vi "CRYRub & Buzz Spreading.vi"(8 "number":i32, 9 "Pp[k]":dbl[](array[numeric]), 10 "Version":i32, 11 "Real matrix":dbl[][](array[numeric])) -> (3 "E2[k]":dbl[](array[numeric]))   [LabVIEW 2013]
panel:
  out "Su[k]":dbl[](array[numeric])
  out "Eline[j,k]":dbl[][](array[numeric])
  out "Eline1[j,k]":dbl[][](array[numeric])
  out "Sl[k]":dbl[](array[numeric])
  out "NormSP[k]":dbl[](array[numeric])
  out "L[k]":dbl[](array[numeric])
  in  "res":dbl
  out "Su[k]":dbl[](array[numeric])
  out "Eline[j,k]":dbl[][](array[numeric])
  out "Eline1[j,k]":dbl[][](array[numeric])
  out "Sl[k]":dbl[](array[numeric])
  out "L[k]":dbl[](array[numeric])
  in  "res":dbl
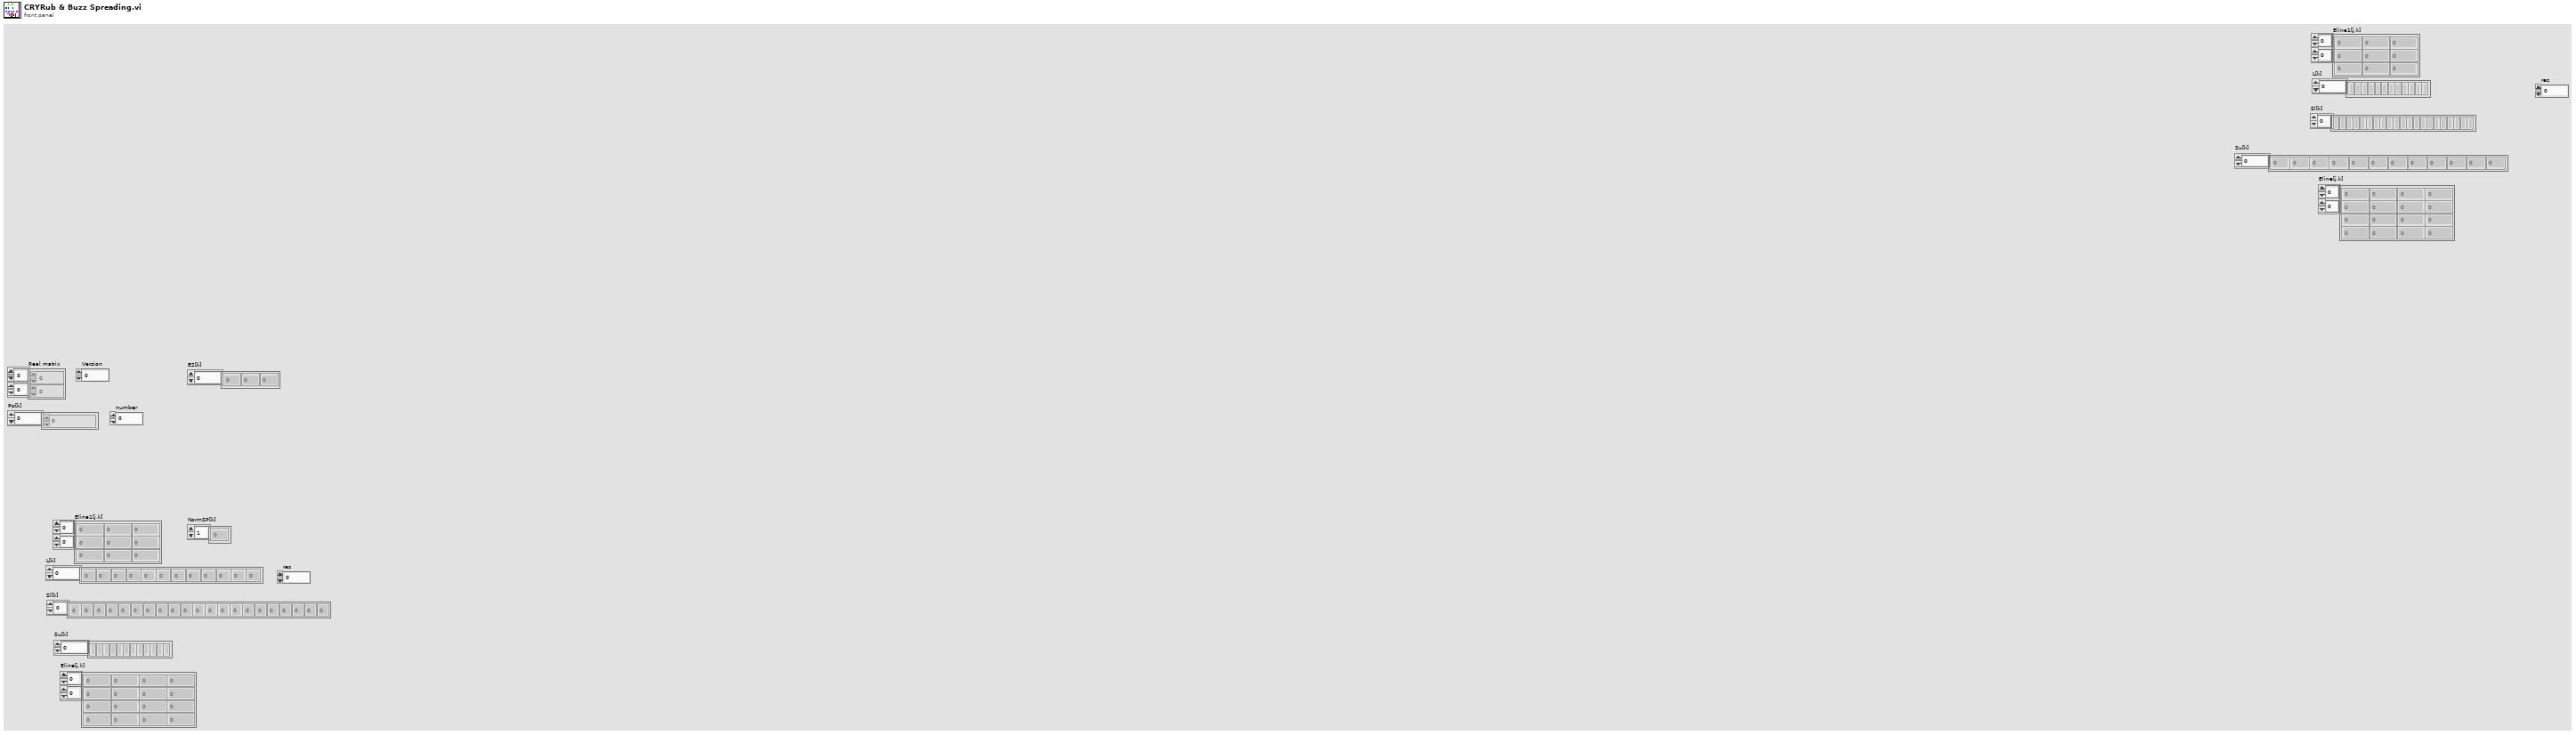
[diagram p1: front panel]
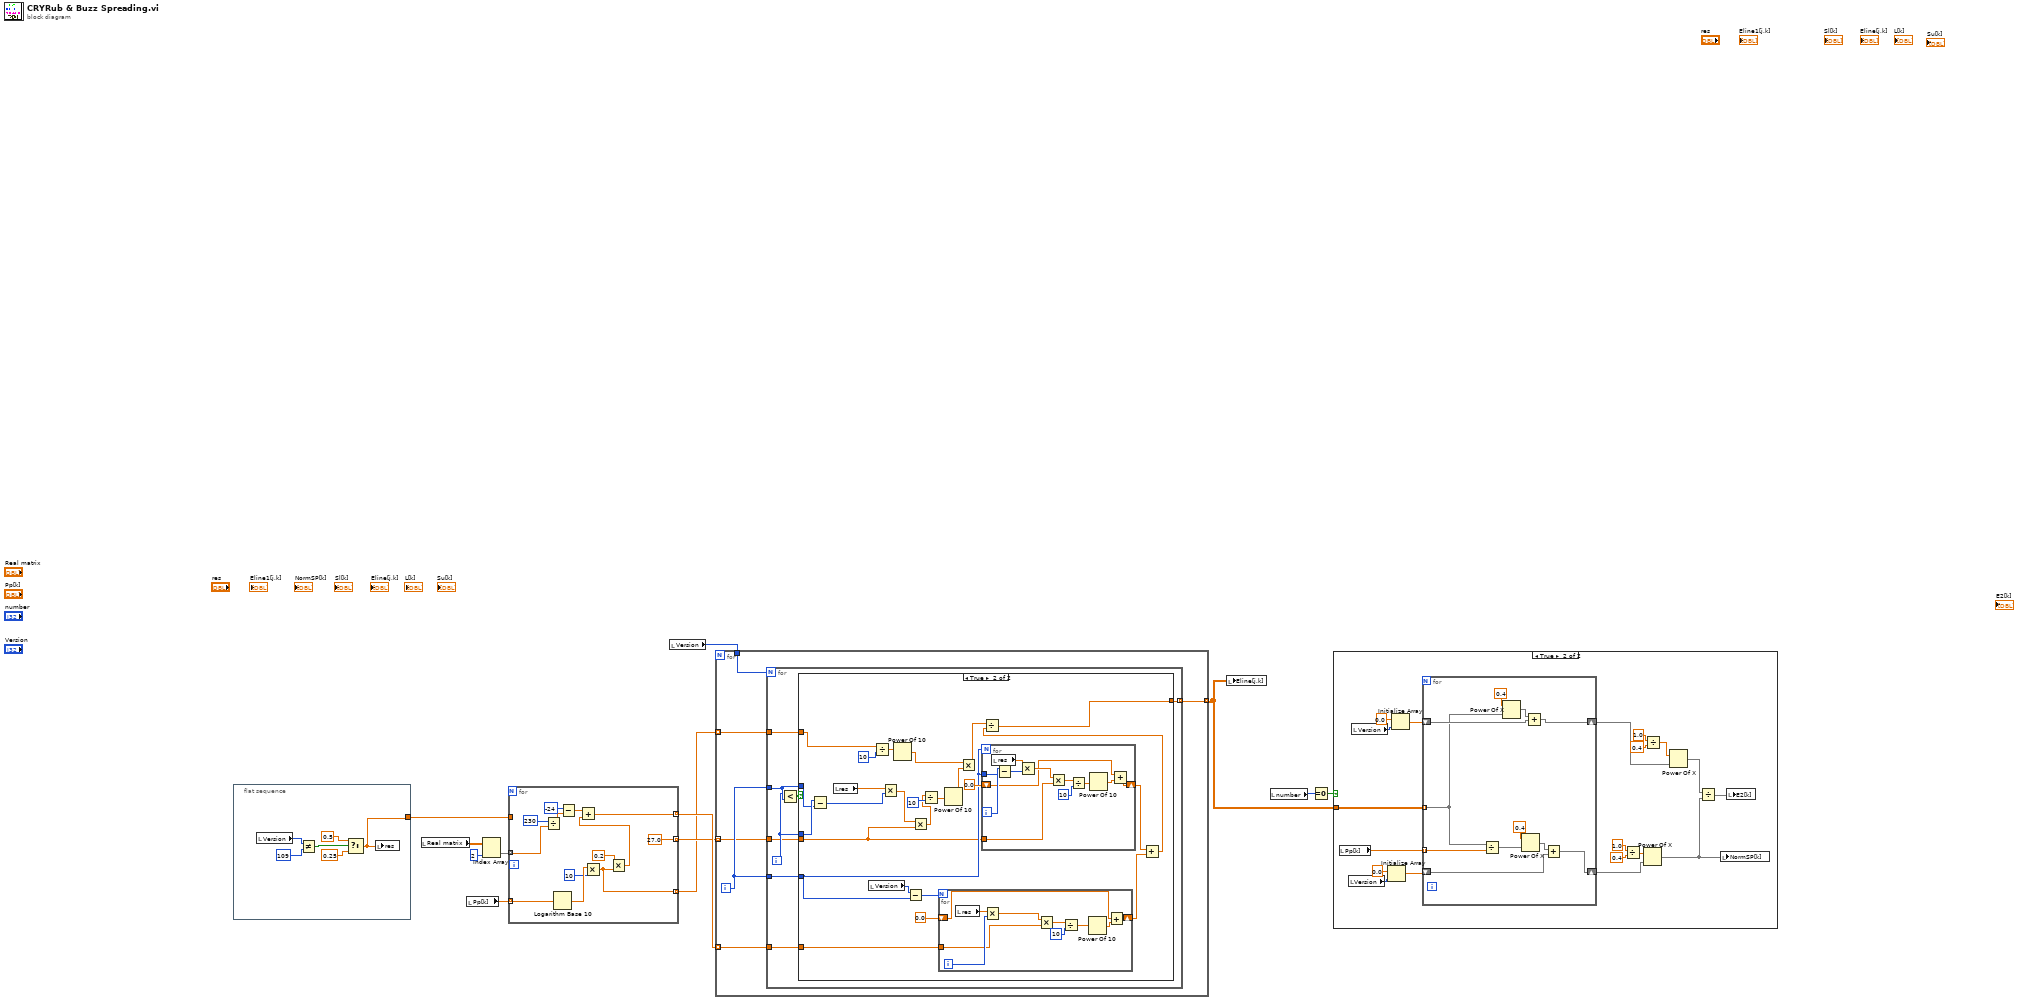
[diagram p0: block diagram]
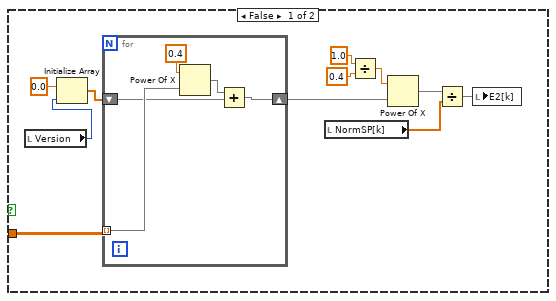
[diagram p2: hidden frame]
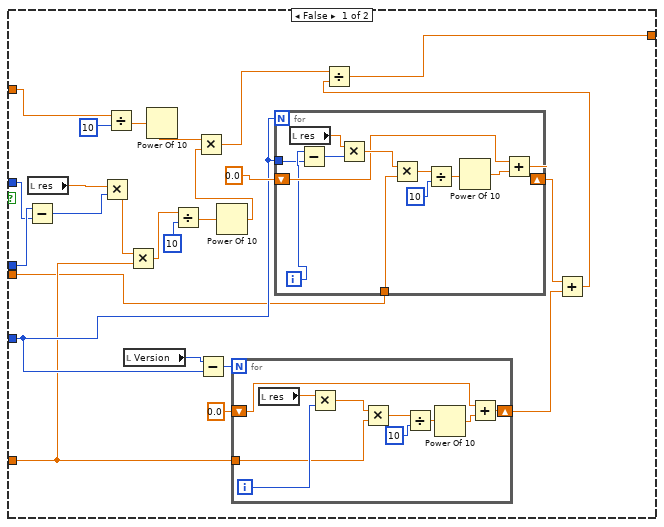
[diagram p3: hidden frame]
diagram:
  n1 = flat-sequence {
    tunnel: [w13] -> w3
    frame #0 {
      n2 = local read "Version"() -> (w17:i32)
      n3 = Not Equal?(x=w17, y=109) -> (x != y?=w16:bool)
      n4 = Select(t=0.5, s=w16, f=0.25) -> (s? t:f=w13:dbl)
      n5 = local write "res"(w13) -> ()
    }
  }
  n6 = local read "Real matrix"() -> (w8:dbl[][])
  n7 = local read "Pp[k]"() -> (w1:dbl[])
  n8 = Index Array(array=w8, index (col)=2 ("disabled index (col)")) -> (element=w6:dbl[])  [unwired: 1 in]
  n9 = for {
    tunnel: w1 -> [w23] mode=indexing
    tunnel: w6 -> [w19] mode=indexing
    tunnel: [w22] -> w10 mode=indexing
    tunnel: [27.0] -> w9 mode=indexing
    tunnel: [w20] -> w2 mode=indexing
    tunnel: w3 -> [_]
    n10 = Divide(x=230, y=w19) -> (x/y=w28:dbl)
    n11 = Logarithm Base 10(1:w23) -> (0:w31:dbl)
    n12 = Subtract(x=-24, y=w28) -> (x-y=w25:dbl)
    n13 = Multiply ("Multiply.vi")(x=w31, y=10) -> (x*y=w20:dbl)
    n14 = Multiply ("Multiply.vi")(x=0.2, y=w20) -> (x*y=w24:dbl)
    n15 = Add ("Add.vi")(x=w25, y=w24) -> (x+y=w22:dbl)
  }
  n16 = local read "Version"() -> (w11:i32)
  n17 = for {
    tunnel: w11 -> [w37]
    tunnel: w10 -> [w36] mode=indexing
    tunnel: w2 -> [w34] mode=indexing
    tunnel: [w32] -> w12 mode=indexing
    tunnel: w9 -> [w33] mode=indexing
    i -> [w35]
    n18 = for {
      N: w37 -> [_]
      tunnel: w35 -> [w44]
      tunnel: w35 -> [w43]
      tunnel: w36 -> [w41]
      tunnel: w34 -> [w40]
      tunnel: [w39] -> w32 mode=indexing
      tunnel: w33 -> [w38]
      i -> [w42]
      n19 = Less?(x=w42, y=w44) -> (x < y?=w45:bool)
      n20 = case shown="True" w45 {
        tunnel: w44 -> [w59 w105]
        tunnel: w42 -> [w60 w116]
        tunnel: w43 -> [w52 w100]
        tunnel: w41 -> [w48 w94]
        tunnel: w40 -> [w50 w97]
        tunnel: [w49 w96] -> w39
        tunnel: w38 -> [w47 w95]
        frame False {
          n21 = Subtract(x=w60, y=w59) -> (x-y=w69:i32)
          n22 = local read "res"() -> (w46:dbl)
          n23 = Multiply(x=w46, y=w69) -> (x*y=w55:dbl)
          n24 = Divide(x=w50, y=10) -> (x/y=w65:dbl)
          n25 = local read "Version"() -> (w51:i32)
          n26 = Multiply ("Multiply.vi")(x=w55, y=w48) -> (x*y=w54:dbl)
          n27 = Power Of 10(x=w65) -> (10^x=w64:dbl)
          n28 = Divide(x=w54, y=10) -> (x/y=w67:dbl)
          n29 = Subtract(x=w51, y=w52) -> (x-y=w63:i32)
          n30 = Power Of 10(x=w67) -> (10^x=w66:dbl)
          n31 = Multiply ("Multiply.vi")(x=w64, y=w66) -> (x*y=w61:dbl)
          n32 = for {
            N: w63 -> [_]
            shift-right: [w74] -> w62
            shift-left: 0.0 ("10^x") -> [w71]
            tunnel: w48 -> [w73]
            i -> [w80]
            n33 = local read "res"() -> (w72:dbl)
            n34 = Multiply ("Multiply.vi")(x=w72, y=w80) -> (x*y=w79:dbl)
            n35 = Multiply ("Multiply.vi")(x=w79, y=w73) -> (x*y=w78:dbl)
            n36 = Divide(x=w78, y=10) -> (x/y=w76:dbl)
            n37 = Power Of 10(x=w76) -> (10^x=w75:dbl)
            n38 = Add ("Add.vi")(x=w71, y=w75) -> (x+y=w74:dbl)
          }
          n39 = for {
            N: w52 -> [_]
            tunnel: w52 -> [w83]
            shift-right: [w85] -> w58
            shift-left: 0.0 ("10^x") -> [w86]
            tunnel: w47 -> [w82]
            i -> [w84]
            n40 = local read "res"() -> (w81:dbl)
            n41 = Subtract(x=w84, y=w83) -> (x-y=w92:i32)
            n42 = Multiply ("Multiply.vi")(x=w81, y=w92) -> (x*y=w91:dbl)
            n43 = Multiply ("Multiply.vi")(x=w91, y=w82) -> (x*y=w90:dbl)
            n44 = Divide(x=w90, y=10) -> (x/y=w88:dbl)
            n45 = Power Of 10(x=w88) -> (10^x=w87:dbl)
            n46 = Add ("Add.vi")(x=w86, y=w87) -> (x+y=w85:dbl)
          }
          n47 = Add ("Add.vi")(x=w58, y=w62) -> (x+y=w53:dbl)
          n48 = Divide(x=w61, y=w53) -> (x/y=w49:dbl)
        }
        frame True {
          n49 = Subtract(x=w116, y=w105) -> (x-y=w115:i32)
          n50 = local read "res"() -> (w93:dbl)
          n51 = local read "Version"() -> (w98:i32)
          n52 = Divide(x=w97, y=10) -> (x/y=w111:dbl)
          n53 = Multiply(x=w93, y=w115) -> (x*y=w104:dbl)
          n54 = Power Of 10(x=w111) -> (10^x=w110:dbl)
          n55 = Subtract(x=w98, y=w100) -> (x-y=w109:i32)
          n56 = Multiply ("Multiply.vi")(x=w104, y=w95) -> (x*y=w103:dbl)
          n57 = Divide(x=w103, y=10) -> (x/y=w113:dbl)
          n58 = for {
            N: w109 -> [_]
            shift-right: [w121] -> w107
            shift-left: 0.0 -> [w120]
            tunnel: w94 -> [w119]
            i -> [w127]
            n59 = local read "res"() -> (w118:dbl)
            n60 = Multiply(x=w118, y=w127) -> (x*y=w126:dbl)
            n61 = Multiply ("Multiply.vi")(x=w126, y=w119) -> (x*y=w125:dbl)
            n62 = Divide(x=w125, y=10) -> (x/y=w123:dbl)
            n63 = Power Of 10(x=w123) -> (10^x=w122:dbl)
            n64 = Add ("Add.vi")(x=w120, y=w122) -> (x+y=w121:dbl)
          }
          n65 = Power Of 10(x=w113) -> (10^x=w112:dbl)
          n66 = Multiply ("Multiply.vi")(x=w110, y=w112) -> (x*y=w106:dbl)
          n67 = for {
            N: w100 -> [_]
            tunnel: w100 -> [w138]
            shift-right: [w133] -> w108
            shift-left: 0.0 -> [w130]
            tunnel: w95 -> [w129]
            i -> [w139]
            n68 = local read "res"() -> (w128:dbl)
            n69 = Subtract(x=w139, y=w138) -> (x-y=w137:i32)
            n70 = Multiply(x=w128, y=w137) -> (x*y=w136:dbl)
            n71 = Multiply ("Multiply.vi")(x=w136, y=w129) -> (x*y=w135:dbl)
            n72 = Divide(x=w135, y=10) -> (x/y=w132:dbl)
            n73 = Power Of 10(x=w132) -> (10^x=w131:dbl)
            n74 = Add ("Add.vi")(x=w130, y=w131) -> (x+y=w133:dbl)
          }
          n75 = Add ("Add.vi")(x=w108, y=w107) -> (x+y=w101:dbl)
          n76 = Divide(x=w106, y=w101) -> (x/y=w96:dbl)
        }
      }
    }
  }
  n77 = local write "Eline[j,k]"(w12) -> ()
  n78 = local read "number"() -> (w5:i32)
  n79 = Equal To 0?(x=w5) -> (x = 0?=w4:bool)
  n80 = case shown="True" w4 {
    tunnel: w12 -> [w150 w174]
    frame False {
      n81 = local read "Version"() -> (w140:i32)
      n82 = Initialize Array(0.0 ("element"), w140) -> (w142:dbl[])
      n83 = for {
        tunnel: w150 -> [w153] mode=indexing
        shift-right: [w151] -> w147
        shift-left: w142 -> [w152]
        n84 = Power Of X(1:w153, 2:0.4) -> (0:w155:dbl[])
        n85 = Add(x=w155, y=w152) -> (x+y=w151:dbl[])
      }
      n86 = local read "NormSP[k]"() -> (w148:dbl[])
      n87 = Divide(x=1.0, y=0.4) -> (x/y=w144:dbl)
      n88 = Power Of X(1:w147, 2:w144) -> (0:w143:dbl[])
      n89 = Divide(x=w143, y=w148) -> (x/y=w149:dbl[])
      n90 = local write "E2[k]"(w149) -> ()
    }
    frame True {
      n91 = local read "Pp[k]"() -> (w156:dbl[])
      n92 = local read "Version"() -> (w159:i32)
      n93 = local read "Version"() -> (w165:i32)
      n94 = Initialize Array(0.0 ("element"), w159) -> (w158:dbl[])
      n95 = Initialize Array(0.0 ("element"), w165) -> (w157:dbl[])
      n96 = for {
        tunnel: w156 -> [w181] mode=indexing
        tunnel: w174 -> [w176] mode=indexing
        shift-right: [w182] -> w161
        shift-left: w158 -> [w184]
        shift-right: [w177] -> w166
        shift-left: w157 -> [w179]
        n97 = Divide(x=w176, y=w181) -> (x/y=w175:dbl[])
        n98 = Power Of X(1:w176, 2:0.4) -> (0:w178:dbl[])
        n99 = Power Of X(1:w175, 2:0.4) -> (0:w180:dbl[])
        n100 = Add(x=w178, y=w179) -> (x+y=w177:dbl[])
        n101 = Add(x=w180, y=w184) -> (x+y=w182:dbl[])
      }
      n102 = Divide(x=1.0, y=0.4) -> (x/y=w167:dbl)
      n103 = Power Of X(1:w161, 2:w167) -> (0:w163:dbl[])
      n104 = Divide(x=1.0, y=0.4) -> (x/y=w171:dbl)
      n105 = Power Of X(1:w166, 2:w171) -> (0:w170:dbl[])
      n106 = Divide(x=w170, y=w163) -> (x/y=w162:dbl[])
      n107 = local write "NormSP[k]"(w163) -> ()
      n108 = local write "E2[k]"(w162) -> ()
    }
  }
